vi "Roll detection TEST.vi"() -> ()   [LabVIEW 2018]
uses:
  <vilib>/myRIO/Instrument Drivers/Onboard Devices/Accelerometer/typedefs/Accelerometer Reference.ctl
  <vilib>/myRIO/Common/Instrument Driver Framework/Utilities/typedefs/myRIO Generic Hardware Reference.ctl
  <vilib>/myRIO/Common/Instrument Driver Framework/Utilities/typedefs/Hardware Version Enum.ctl
  <vilib>/myRIO/Common/Instrument Driver Framework/Utilities/typedefs/myRIO v1.0 Reference.ctl
  <vilib>/myRIO/Common/Instrument Driver Framework/Utilities/typedefs/Generic FPGA Reference.ctl
  <vilib>/myRIO/Common/Instrument Driver Framework/myRIO v1.0/Accelerometer/typedefs/Accelerometer Channels List.ctl
  <vilib>/myRIO/Common/Instrument Driver Framework/myRIO v1.0/Accelerometer/typedefs/Accelerometer Channels Enum.ctl
  <vilib>/userdefined/High Color/nirio_resource_hc.ctl
  <vilib>/myRIO/Common/Instrument Driver Framework/myRIO v1.0/Accelerometer/vis/myRIO v1.1 Open Accelerometer.vi
  <vilib>/myRIO/Common/Instrument Driver Framework/Utilities/vis/Validate Channels.vi
  <vilib>/myRIO/Common/Instrument Driver Framework/myRIO v1.0/Accelerometer/vis/myRIO v1.0 Reserve Accelerometer.vi
  <vilib>/myRIO/Common/Instrument Driver Framework/myRIO v1.0/Accelerometer/vis/myRIO v1.0 Close Accelerometer.vi
  <vilib>/myRIO/Common/Instrument Driver Framework/myRIO v1.0/Resource Manager/vis/myRIO v1.0 Reserve Channel List.vi
  <vilib>/myRIO/Common/Instrument Driver Framework/myRIO v1.0/Accelerometer/vis/myRIO v1.0 Build MUX Configuration Accelerometer.vi
  <vilib>/myRIO/Common/Instrument Driver Framework/myRIO v1.0/Accelerometer/vis/myRIO v1.0 Unreserve Accelerometer.vi
  <vilib>/myRIO/Common/Instrument Driver Framework/myRIO v1.0/Resource Manager/vis/myRIO v1.0 Reserve Channel.vi
  <vilib>/myRIO/Common/Instrument Driver Framework/myRIO v1.0/Resource Manager/vis/myRIO v1.0 Unreserve Channel.vi
  <vilib>/myRIO/Common/Instrument Driver Framework/myRIO v1.0/Resource Manager/vis/myRIO v1.0 Unreserve Channel List.vi
  <vilib>/myRIO/Common/Instrument Driver Framework/myRIO v1.0/Resource Manager/vis/myRIO v1.0 Build Mutex Name.vi
  <vilib>/Utility/VariantDataType/GetNumericInfo.vi
  <vilib>/Utility/error.llb/Error Cluster From Error Code.vi
  <vilib>/myRIO/Common/Instrument Driver Framework/myRIO v1.0/myRIO v1.1 Open.vi
  <vilib>/myRIO/Common/Instrument Driver Framework/myRIO v1.0/Accelerometer/vis/myRIO v1.0 Get Scaling Constant Accelerometer.vi
  <vilib>/myRIO/Common/Instrument Driver Framework/Utilities/vis/IO Manager.vi
  <vilib>/myRIO/Common/Instrument Driver Framework/Utilities/vis/Configuration Manager.vi
  <vilib>/myRIO/Common/Instrument Driver Framework/myRIO v1.0/myRIO v1.0 Close.vi
  <vilib>/myRIO/Common/Instrument Driver Framework/myRIO v1.0/Accelerometer/vis/myRIO v1.0 Read Accelerometer.vi
  <vilib>/myRIO/Instrument Drivers/Onboard Devices/Accelerometer/vis/myRIO Accelerometer Open.xnode
  <vilib>/myRIO/Instrument Drivers/Onboard Devices/Accelerometer/Accelerometer.lvlib
panel:
  out "Alarm":bool
  in  "Grounded?":bool
  in  "stop":bool
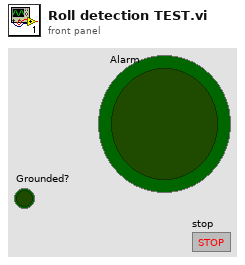
[diagram p1: front panel]
types:
  T1 = typedef "Accelerometer.lvlib/Accelerometer Reference.ctl" = cluster{"myRIO Reference":T2, "Accelerometer Channels List":T6, "LSB Weight":dbl}
  T2 = typedef "myRIO Generic Hardware Reference.ctl" = cluster{"myRIO Model":T3, "myRIO Hardware Reference":T4}
  T3 = typedef "Hardware Version Enum.ctl" = enum16{"Unknown", "myRIO-1900", "myRIO-1950", "roboRIO", "NI ELVIS RIO CM", "ELVIS III"}
  T4 = typedef "myRIO v1.0 Reference.ctl" = cluster{"Generic FPGA Reference":T5, "Allow multiple opens":bool}
  T5 = typedef "Generic FPGA Reference.ctl" = refnum<k20>
  T6 = typedef "Accelerometer Channels List.ctl" = T7[]
  T7 = typedef "Accelerometer Channels Enum.ctl" = enum16{"Not Connected", "X-Axis", "Y-Axis", "Z-Axis"}
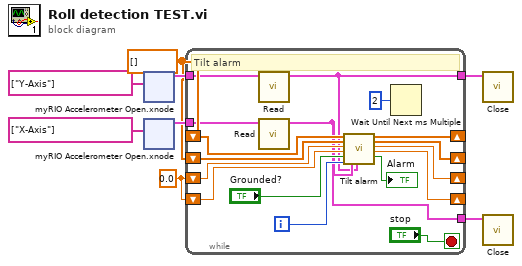
[diagram p0: block diagram]
diagram:
  w1 = 0.0 ("X-Stored-Shift-out")
  w2 = dbl[] [] ("X-Array-Shift-out")
  n1 = xnode "myRIO Accelerometer Open.xnode"("Channel Names"=tag[] ["Y-Axis"]) -> ("Accelerometer Ref Out"=w5:T1)  [unwired: 2 in, 1 out]
  n2 = xnode "myRIO Accelerometer Open.xnode"("Channel Names"=tag[] ["X-Axis"]) -> ("Accelerometer Ref Out"=w7:T1)  [unwired: 2 in, 1 out]
  n3 = while {
    shift-right: [w13] -> _
    shift-left: w2 -> [w22]
    shift-right: [w12] -> _
    shift-left: w2 -> [w21]
    shift-right: [w11] -> _
    shift-left: w1 -> [w20]
    shift-right: [w10] -> _
    shift-left: w1 -> [w19]
    tunnel: [w16] -> w8
    tunnel: w7 -> [w24]
    tunnel: w5 -> [w23]
    tunnel: [w15] -> w3
    i -> [w17]
    stop <- "stop" stop-if-true
    # "Tilt alarm"
    n4 = call <vilib>:"Read.vi"("Accelerometer Ref In"=w23) -> ("Accelerometer Ref Out"=w15:T1)  [unwired: 8 in, 2 out]
    n5 = call <vilib>:"Read.vi"("Accelerometer Ref In"=w24) -> ("Accelerometer Ref Out"=w16:T1)  [unwired: 8 in, 2 out]
    n6 = call "Tilt alarm.vi"("X-Array-Shift-in"=w22, "Y-Array-Shift-in"=w21, "X-Stored-Shift-in"=w20, "Y-Stored-Shift-in"=w19, "Grounded?"="Grounded?", "Iterations"=w17, "Accelerometer Ref X in"=w16, "Accelerometer Ref Y In"=w15) -> ("X-Array-Shift-out"=w13:dbl[], "Y-Array-Shift-out"=w12:dbl[], "X-Stored-Shift-out"=w11:dbl, "Y-Stored-Shift-out"=w10:dbl, "Alarm"=→"Alarm":bool)  [unwired: 7 in]
    n7 = Wait Until Next ms Multiple(millisecond multiple=u32 2) -> ()  [unwired: 1 out]
  }
  n8 = call <vilib>:"Close.vi"("Accelerometer Ref In"=w3) -> ()  [unwired: 10 in, 1 out]
  n9 = call <vilib>:"Close.vi"("Accelerometer Ref In"=w8) -> ()  [unwired: 10 in, 1 out]
